vi "Unmap and Remove Tag by Channel.vi"(7 "owner ID":string, 8 "error in":errorcluster, 9 "Delete Unmapped Tag? (True)":bool=TRUE, 10 "channel":refnum<class "TBM channel.lvclass">, 11 "engine configuration in":refnum<class "engine configuration.lvclass">) -> (0 "error out":errorcluster, 3 "engine configuration out":refnum<class "engine configuration.lvclass">)   [LabVIEW 2015, in "E2E Tag Exchange editor node.lvclass"]
uses:
  E2E Tag Exchange editor node.lvclass
  <vilib>/NI/Tag Bus Module Framework/channel/TBM channel.lvclass
  <vilib>/NI/Module Execution Interface/Engine Configuration/engine configuration.lvclass
  <vilib>/NI/Tag Bus/tag/tag descriptor.lvclass/tag descriptor.ctl
  <vilib>/NI/Tag Bus/tag/tag descriptor.lvclass
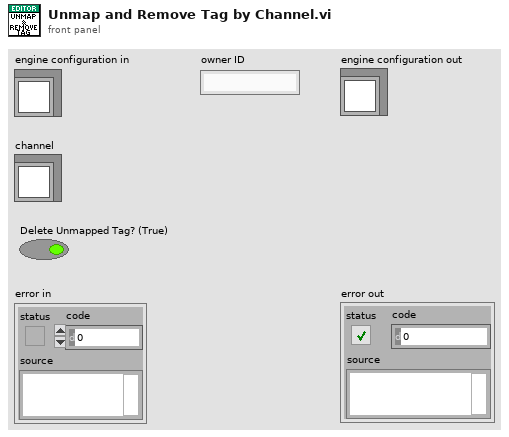
[diagram p1: front panel]
types:
  T1 = typedef "engine configuration.lvclass/unique channel identifier.ctl" = cluster{"channel":string, "module ID":string}
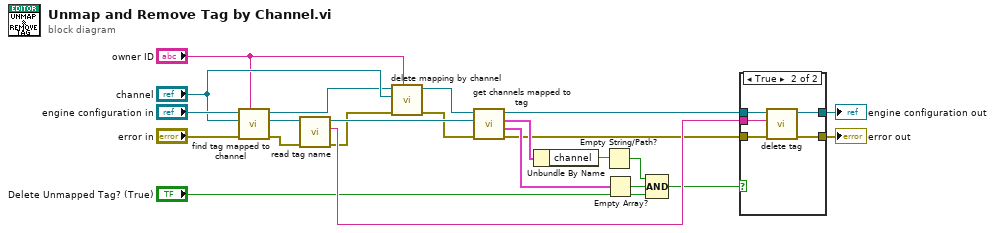
[diagram p0: block diagram]
diagram:
  n1 = call <vilib>:"find tag mapped to channel.vi"("owner"="owner ID", "error in"="error in", "channel"="channel", "engine configuration in"="engine configuration in") -> ("error out"=w15:errorcluster, "tag"=w14:refnum<class "tag descriptor.lvclass">, "engine configuration out"=w5:refnum<class "engine configuration.lvclass">)  [unwired: 5 in]
  n2 = call <vilib>:"read tag name.vi"("error in"=w15, "system tag in"=w14) -> ("error out"=w6:errorcluster, "name"=w12:string, "system tag out"=w13:refnum<class "tag descriptor.lvclass">)  [unwired: 7 in]
  n3 = call <vilib>:"delete mapping by channel.vi"("owner ID"="owner ID", "error in"=w6, "channel"="channel", "engine configuration in"=w5) -> ("error out"=w3:errorcluster, "engine configuration out"=w4:refnum<class "engine configuration.lvclass">)  [unwired: 6 in]
  n4 = call-dynamic "get channels mapped to tag.vi"("error in"=w3, "tag"=w13, "engine configuration in"=w4) -> ("error out"=w2:errorcluster, "readers"=w23:T1[], "writer"=w20:T1, "engine configuration out"=w1:refnum<class "engine configuration.lvclass">)  [unwired: 5 in]
  n5 = Unbundle By Name(w20) -> ("channel"=w19:string)
  n6 = Empty String/Path?(string/path=w19) -> (empty?=w22:bool)
  n7 = Empty Array?(array=w23) -> (empty?=w21:bool)
  n8 = Compound Arithmetic op=AND(w22, w21, "Delete Unmapped Tag? (True)") -> (w9:bool)
  n9 = case shown="True" w9 {
    tunnel: w1 -> [w25 w30]
    tunnel: w12 -> [_ w29]
    tunnel: w2 -> [w24 w28]
    tunnel: [w24 w27] -> w11
    tunnel: [w25 w26] -> w7
    frame False {
    }
    frame True {
      n10 = call-dynamic "delete tag.vi"("error in"=w28, "tag name"=w29, "engine configuration in"=w30) -> ("error out"=w27:errorcluster, "engine configuration out"=w26:refnum<class "engine configuration.lvclass">)  [unwired: 7 in]
    }
  }
  "error out" <- w11
  "engine configuration out" <- w7
